vi "GetXY.vi"(8 "error in (no error)":errorcluster, 11 "connection ID":refnum<k5>) -> (0 "error out":errorcluster, 1 "Y":dbl format="%#_8g", 2 "X":dbl format="%#_8g", 3 "connection ID out":refnum<k5>)   [LabVIEW 2019]
uses:
  <vilib>/regexp/Match Regular Expression.xnode
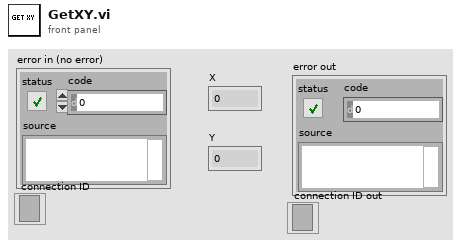
[diagram p1: front panel]
types:
  T1 = enum16{"Standard", "Buffered", "CRLF", "Immediate"}
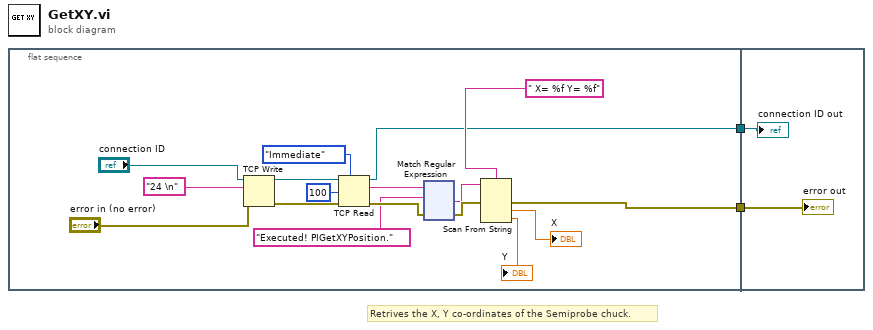
[diagram p0: block diagram]
diagram:
  # "Retrives the X, Y co-ordinates of the Semiprobe chuck."
  n1 = flat-sequence {
    tunnel: [w4] -> w2
    tunnel: [w3] -> w1
    tunnel: w2 -> [w135]
    tunnel: w1 -> [w134]
    frame #0 {
      n2 = TCP Write(connection ID="connection ID", data in="24 \n" ("initial string"), error in (no error)="error in (no error)") -> (connection ID out=w18:refnum<k5>, error out=w19:errorcluster)  [unwired: 1 in, 1 out]
      n3 = TCP Read(connection ID=w18, bytes to read=100, error in (no error)=w19, 7:T1."Immediate" ("mode (standard)")) -> (connection ID out=w3:refnum<k5>, data out=w13:string, error out=w11:errorcluster)  [unwired: 1 in]
      n4 = xnode "Match Regular Expression"("input string"=w13, "regular expression"="Executed! PIGetXYPosition.", "error in"=w11) -> ("after match"=w8:string, "error out"=w10:errorcluster)  [unwired: 3 in, 3 out]
      n5 = Scan From String(format string=" X= %f Y= %f", input string=w8, error in=w10) -> (error out=w4:errorcluster, output 1=→"X":dbl, output 2=→"Y":dbl)  [unwired: 3 in, 2 out]
    }
    frame #1 {
      "error out" <- w135
      "connection ID out" <- w134
    }
  }
